vi "Teleop.vi"(10 "Match Info":T1={"Autonomous Elapsed Seconds"=0.0, "TeleOp Elapsed Seconds"=0.0, "Disabled Elapsed Seconds"=0.0, "Visited Autonomous"=FALSE, "Visited TeleOp"=FALSE, "Visited Disabled"=FALSE, "Autonomous Settings"={"Autonomous Style"=enum."Independent", "VI Refnum"=refnum}}, 11 "Call Context":T2) -> ()   [LabVIEW 2015]
doc: "This VI is called for each TeleOp packet received from the DS where the robot is not disabled. It is often used to read from the joysticks and update I/O or to update setpoints for timed control loops. It should complete and return within 20 milliseconds or it may miss DS packets."
uses:
  <vilib>/Rock Robotics/WPI/DriverStation/WPI_DriverStationDerivedRobotMode.ctl
  <vilib>/Rock Robotics/WPI/DriverStation/WPI_DriverStationMatch Info.ctl
  <vilib>/Rock Robotics/WPI/Utilities/WPI_GetSetVariantRefNum.vi
  <vilib>/Rock Robotics/Network Tables/NT Write Numeric Array.vi
  <vilib>/Rock Robotics/Network Tables/NT Read Boolean.vi
  <vilib>/Rock Robotics/Network Tables/NT Write Boolean.vi
  <vilib>/Rock Robotics/Network Tables/NT Write Number.vi
  <vilib>/Rock Robotics/Network Tables/NT Read Number.vi
  <vilib>/Rock Robotics/Network Tables/NT Write Boolean Array.vi
panel:
  out "Low Switch":bool
  out "High Switch":bool
  out "POT Sensor Meter":dbl(knob) scale=78.0..98.0
  out "POT Sensor Value":dbl
  out "Sample Slider 0":dbl(slide) scale=0.0..5.0
  out "Sample Boolean 1":bool
  out "Sample Boolean 0":bool
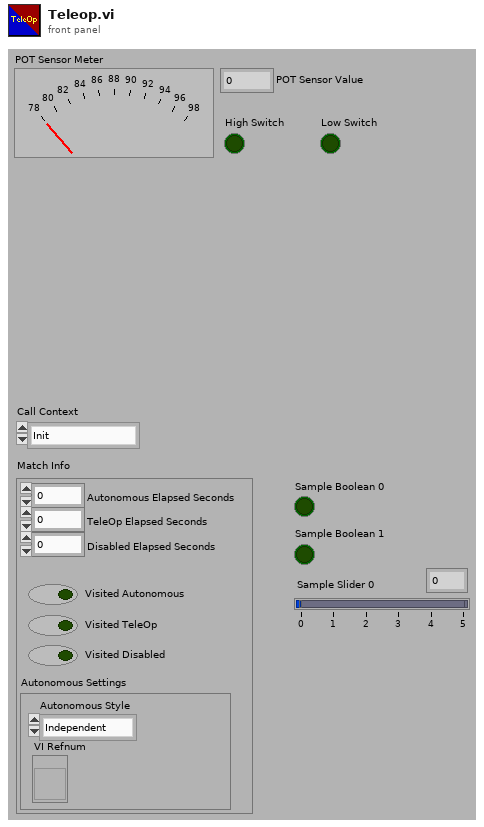
[diagram p1: front panel]
types:
  T1 = typedef "WPI_DriverStationMatch Info.ctl" = cluster{"Autonomous Elapsed Seconds":dbl, "TeleOp Elapsed Seconds":dbl, "Disabled Elapsed Seconds":dbl, "Visited Autonomous":bool, "Visited TeleOp":bool, "Visited Disabled":bool, "Autonomous Settings":cluster{"Autonomous Style":enum16{"Iterative", "Independent"}, "VI Refnum":refnum<vi>}}
  T2 = typedef "WPI_DriverStationDerivedRobotMode.ctl" = enum16{"Init", "Execute", "Stop"}
  T3 = typedef "WPI_JoystickDevRef.ctl" = cluster{"Device":T4}
  T4 = typedef "WPI_JoystickDeviceEnum.ctl" = enum16{"USB 0", "USB 1", "USB 2", "USB 3", "USB 4", "USB 5"}
  T5 = typedef "WPI_SwitchDevRef.ctl" = cluster{"DevStatus":errorcluster, "DIO Channel":T6, "CntIndex":T7, "Normally Closed":bool}
  T6 = typedef "FPGA_DIOChannel.ctl" = enum8{"DIO 0", "DIO 1", "DIO 2", "DIO 3", "DIO 4", "DIO 5", "DIO 6", "DIO 7", "DIO 8", "DIO 9", "DIO MXP 0", "DIO MXP 1", "DIO MXP 2", "DIO MXP 3", "DIO MXP 4", "DIO MXP 5", "DIO MXP 6", "DIO MXP 7", "DIO MXP 8", "DIO MXP 9", "DIO MXP 10", "DIO MXP 11", "DIO MXP 12", "DIO MXP 13", "DIO MXP 14", "DIO MXP 15", "Invalid"}
  T7 = typedef "FPGA_CounterCtrSystemIndex.ctl" = enum8{"Ctr 0", "Ctr 1", "Ctr 2", "Ctr 3", "Ctr 4", "Ctr 5", "Ctr 6", "Ctr 7", "Invalid"}
  T8 = typedef "WPI_PotentiometerDevRef.ctl" = cluster{"DevStatus":errorcluster, "Analog Channel":T9, "Invert Output":bool}
  T9 = typedef "FPGA_AIChannel.ctl" = enum8{"AI 0", "AI 1", "AI 2", "AI 3", "AI MXP 0", "AI MXP 1", "AI MXP 2", "AI MXP 3", "Invalid"}
  T10 = cluster{"Axes[0]":dbl, "Axes[1]":dbl, "Axes[2]":dbl, "Axes[3]":dbl, "Axes[4]":dbl, "Axes[5]":dbl, "Axes[6]":dbl, "Axes[7]":dbl, "Axes[8]":dbl}
  T11 = typedef "WPI_RobotDriveDevRef.ctl" = cluster{"DevStatus":errorcluster, "Motors[]":T12[], "Square Inputs":bool, "Max Output":dbl}
  T12 = typedef "WPI_MotorControlDeviceRef.ctl" = cluster{"DeviceStatus":errorcluster, "Type":T13, "PWM":cluster{"PWM Channel":T14, "DeadBand":T15}, "CAN":cluster{"Device Number":u8, "Control Mode":T16, "Semaphore":T17, "Max Vout":dbl, "TalonSRX Control Mode":T18}, "Invert":bool}
  T13 = typedef "WPI_MotorControlType.ctl" = enum16{"PWM", "CAN", "CANTalonSRX"}
  T14 = typedef "FPGA_DIOPWMChannel.ctl" = enum8{"PWM 0", "PWM 1", "PWM 2", "PWM 3", "PWM 4", "PWM 5", "PWM 6", "PWM 7", "PWM 8", "PWM 9", "PWM MXP 0", "PWM MXP 1", "PWM MXP 2", "PWM MXP 3", "PWM MXP 4", "PWM MXP 5", "PWM MXP 6", "PWM MXP 7", "PWM MXP 8", "PWM MXP 9", "Invalid"}
  T15 = typedef "WPI_PWMDeadband.ctl" = cluster{"Name":string, "maxPositivePwm":i32, "minPositivePwm":i32, "centerPwm":i32, "maxNegativePwm":i32, "minNegativePwm":i32, "angularRange":u16}
  T16 = typedef "WPI_CANJaguar_ControlMode.ctl" = enum8{"Percent VBus", "Current", "Speed", "Position", "Voltage"}
  T17 = typedef "Semaphore RefNum" = refnum<k1>
  T18 = typedef "WPI_CANTalonSRX_APIControlMode.ctl" = enum8{"Percent VBus", "Speed", "Position", "Slave", "Unchanged / Invalid", "Voltage Compensation", "Current", "Motion Profile"}
  T19 = cluster{"Buttons[0]":bool, "Buttons[1]":bool, "Buttons[2]":bool, "Buttons[3]":bool, "Buttons[4]":bool, "Buttons[5]":bool, "Buttons[6]":bool, "Buttons[7]":bool, "Buttons[8]":bool}
  T20 = typedef "WPI_ServoDeviceRef.ctl" = cluster{"DeviceStatus":errorcluster, "PWM Channel":T14, "DeadBand":T15}
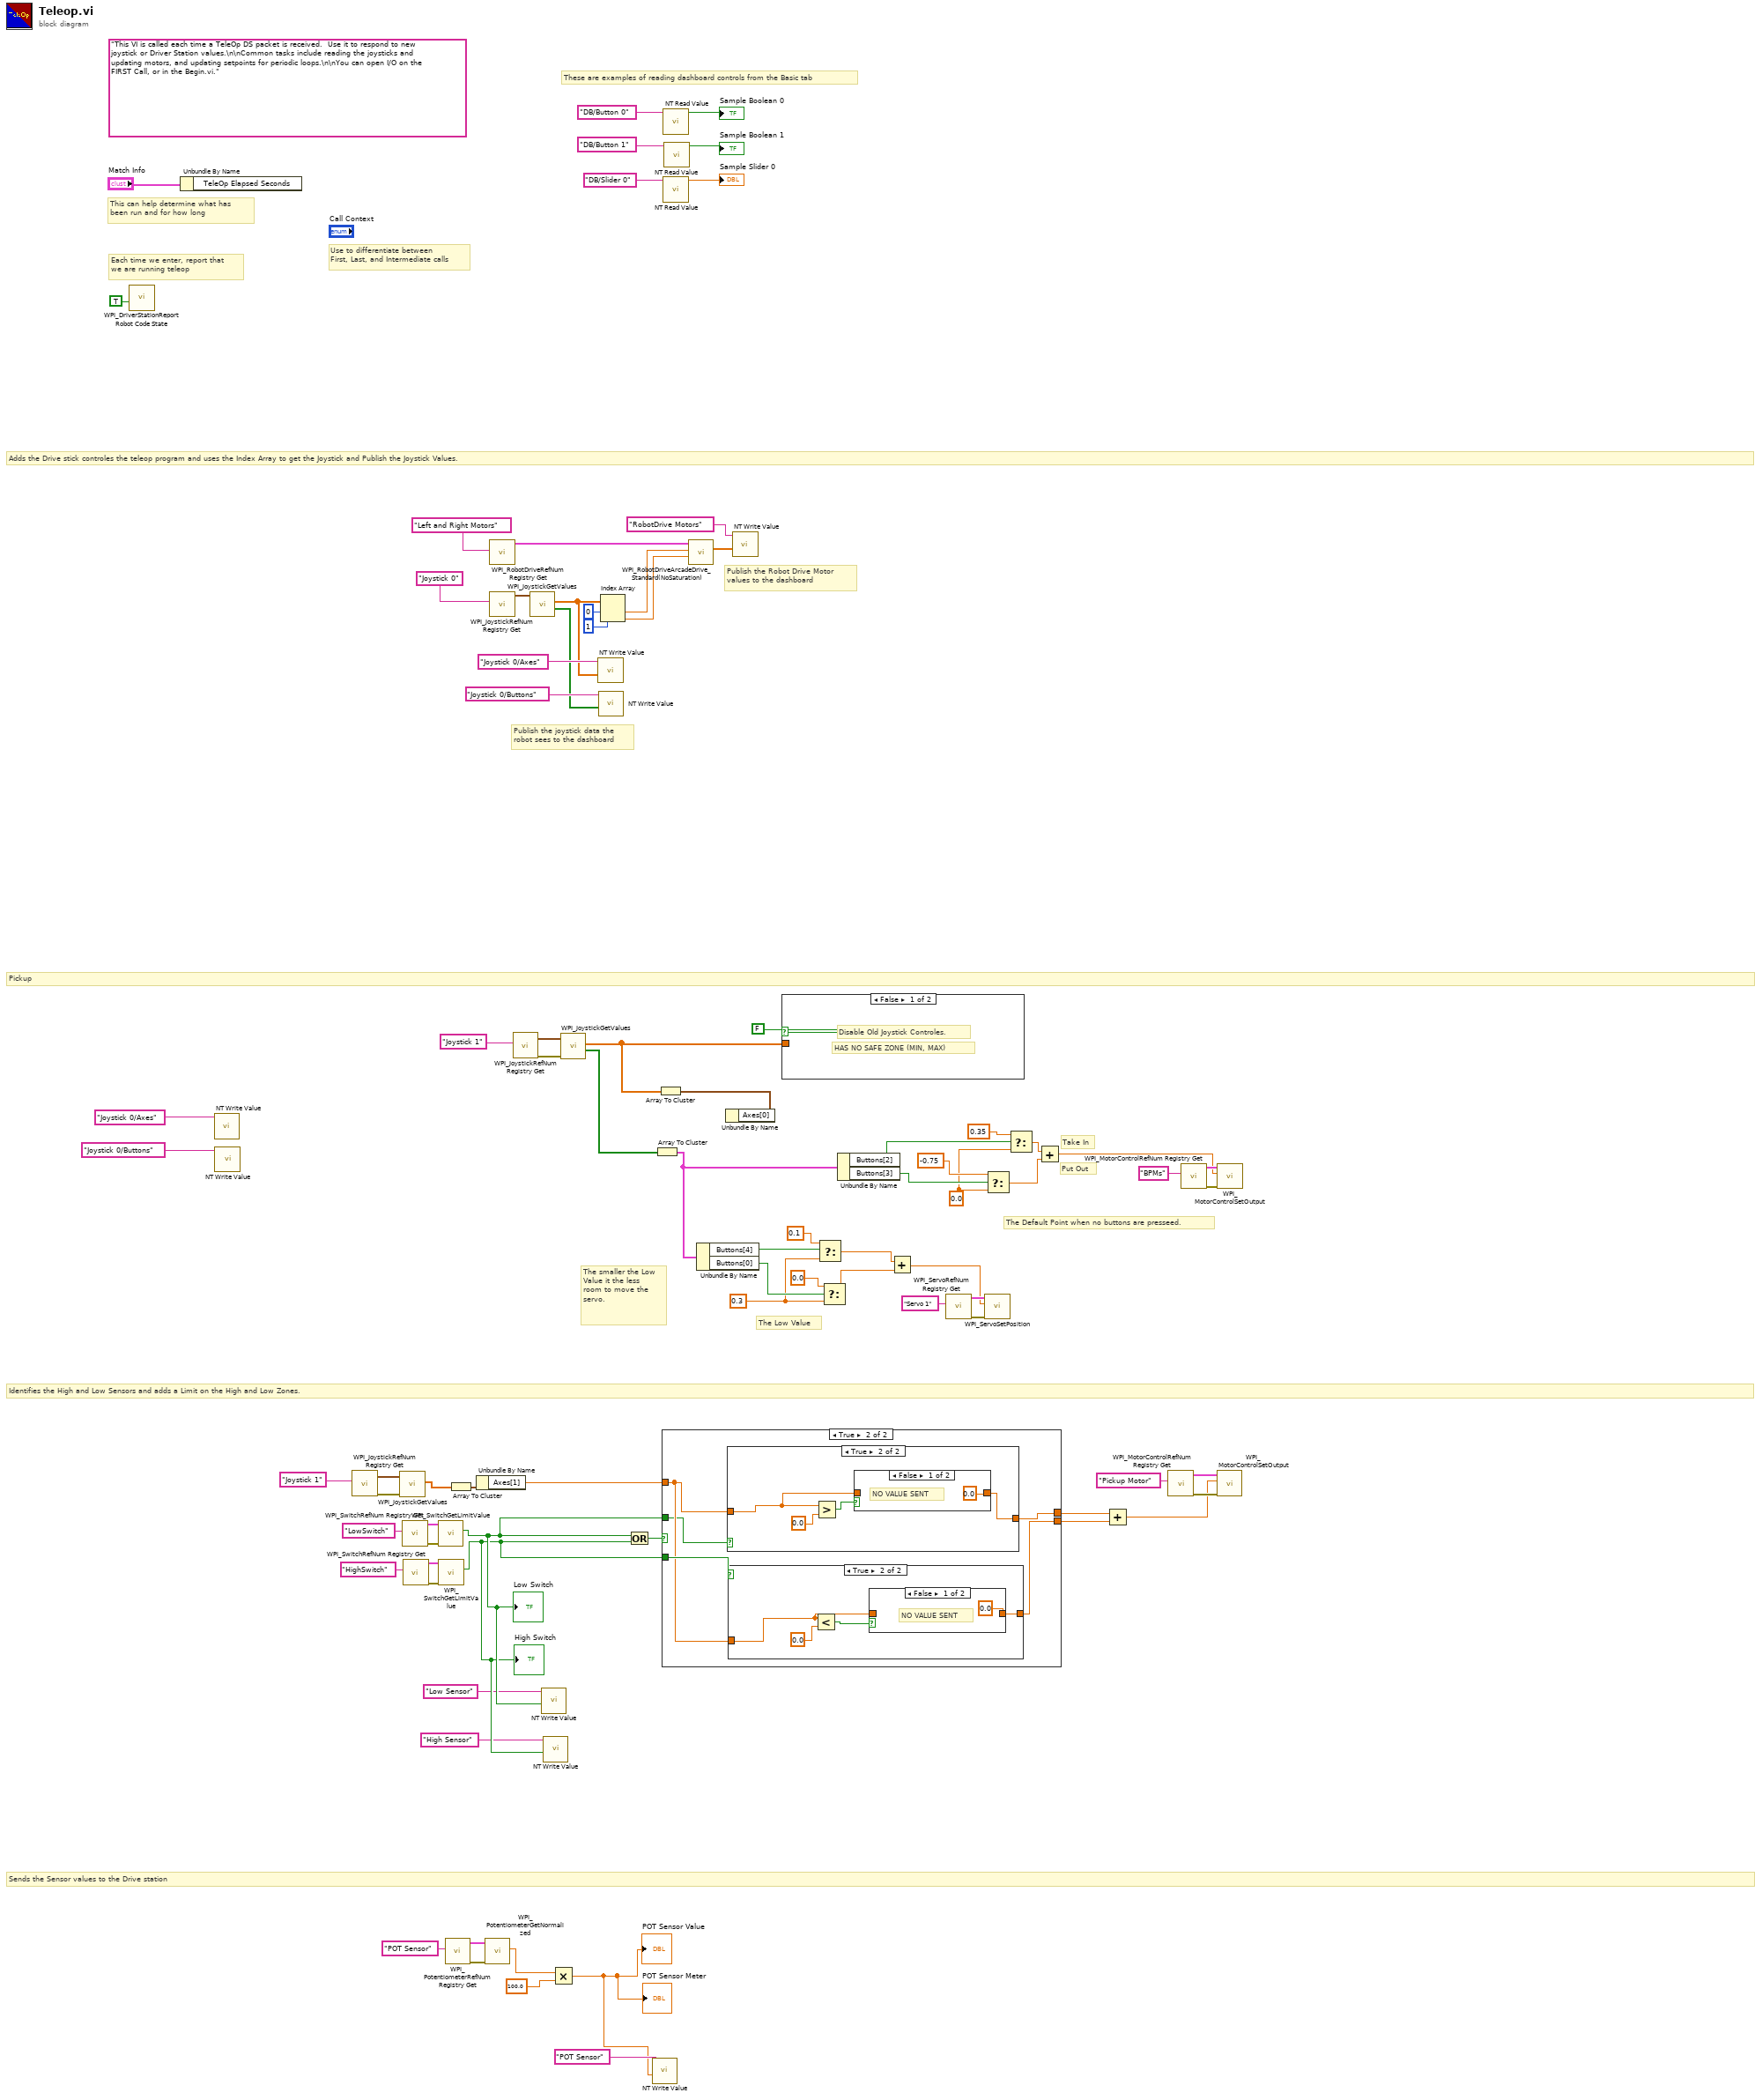
[diagram p0: block diagram]
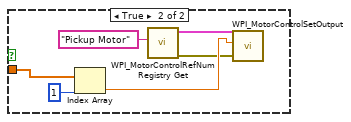
[diagram p2: hidden frame]
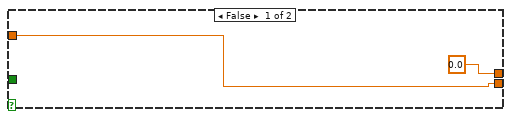
[diagram p3: hidden frame]
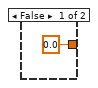
[diagram p4: hidden frame]
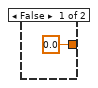
[diagram p6: hidden frame]
diagram:
  w3 = 0.3 ("f")
  w1 = 0.0 ("f")
  (unwired) "This VI is called each time a TeleOp DS packet is received.  Use it to respond to new joystick or Driver Station values.\n\nCommon tasks include reading the joysticks and updating motors, and updating setpoints for periodic loops.\n\nYou can open I/O on the FIRST Call, or in the Begin.vi."
  # "Adds the Drive stick controles the teleop program and uses the Index Array to get the Joystick and Publish the Joystick Values."
  # "Sends the Sensor values to the Drive station"
  # "Identifies the High and Low Sensors and adds a Limit on the High and Low Zones."
  # "The Default Point when no buttons are presseed."
  # "The smaller the Low Value it the less room to move the servo."
  # "The Low Value"
  # "Put Out"
  # "Take In"
  # "Pickup"
  # "These are examples of reading dashboard controls from the Basic tab"
  # "Publish the Robot Drive Motor\nvalues to the dashboard"
  # "Publish the joystick data the\nrobot sees to the dashboard"
  # "Each time we enter, report that\nwe are running teleop"
  # "Use to differentiate between\nFirst, Last, and Intermediate calls"
  # "This can help determine what has\nbeen run and for how long"
  n1 = call <vilib>:"WPI_DriverStationReport Robot Code State.vi"("TeleOp"=TRUE ("Autonomous")) -> ()  [unwired: 10 in, 1 out]
  n2 = Unbundle By Name("Match Info") -> ()  [unwired: 1 out]
  n3 = call-poly <vilib>:"NT Write Value.vi"("Name"="Joystick 0/Axes") -> ()  [unwired: 10 in, 1 out]
  n4 = call-poly <vilib>:"NT Write Value.vi"("Name"="Joystick 0/Buttons") -> ()  [unwired: 10 in, 1 out]
  n5 = call <vilib>:"WPI_JoystickRefNum Registry Get.vi"("refnum name"="Joystick 1") -> ("error out"=w37:errorcluster, "JoystickDevRef"=w38:T3)  [unwired: 9 in]
  n6 = call <vilib>:"WPI_JoystickGetValues.vi"("error in (no error)"=w37, "JoystickDevRef"=w38) -> ("Axes"=w36:dbl[])  [unwired: 5 in, 4 out]
  n7 = call <vilib>:"WPI_SwitchRefNum Registry Get.vi"("refnum name"="LowSwitch") -> ("error out"=w44:errorcluster, "SwitchDevRef"=w45:T5)  [unwired: 9 in]
  n8 = call <vilib>:"WPI_SwitchRefNum Registry Get.vi"("refnum name"="HighSwitch") -> ("error out"=w41:errorcluster, "SwitchDevRef"=w42:T5)  [unwired: 9 in]
  n9 = call <vilib>:"WPI_SwitchGetLimitValue.vi"("error in (no error)"=w44, "SwitchDevRef"=w45) -> ("Switch Pressed"=w21:bool)  [unwired: 7 in, 2 out]
  "Low Switch" <- w21
  n10 = call <vilib>:"WPI_SwitchGetLimitValue.vi"("error in (no error)"=w41, "SwitchDevRef"=w42) -> ("Switch Pressed"=w20:bool)  [unwired: 7 in, 2 out]
  "High Switch" <- w20
  n11 = call <vilib>:"WPI_PotentiometerRefNum Registry Get.vi"("refnum name"="POT Sensor") -> ("error out"=w25:errorcluster, "PotDevRef"=w24:T8)  [unwired: 9 in]
  n12 = Array To Cluster(array=w36) -> (cluster=w35:T10)
  n13 = Unbundle By Name(w35) -> ("Axes[1]"=w34:dbl)
  n14 = call <vilib>:"WPI_PotentiometerGetNormalized.vi"("error in"=w25, "PotDevRef"=w24) -> ("Normalized Value"=w17:dbl)  [unwired: 7 in, 2 out]
  n15 = call <vilib>:"WPI_RobotDriveRefNum Registry Get.vi"("refnum name"="Left and Right Motors") -> ("RobotDriveDevRef"=w82:T11)  [unwired: 1 in, 9 out]
  n16 = call <vilib>:"WPI_JoystickRefNum Registry Get.vi"("refnum name"="Joystick 0") -> ("JoystickDevRef"=w79:T3)  [unwired: 1 in, 9 out]
  n17 = call <vilib>:"WPI_JoystickRefNum Registry Get.vi"("refnum name"="Joystick 1") -> ("error out"=w61:errorcluster, "JoystickDevRef"=w62:T3)  [unwired: 9 in]
  n18 = call <vilib>:"WPI_JoystickGetValues.vi"("JoystickDevRef"=w79) -> ("Buttons"=w47:bool[], "Axes"=w74:dbl[])  [unwired: 6 in, 3 out]
  n19 = call-poly <vilib>:"NT Write Value.vi"("Boolean"=w21, "Name"="Low Sensor") -> ()  [unwired: 9 in, 1 out]
  n20 = call-poly <vilib>:"NT Write Value.vi"("Boolean"=w20, "Name"="High Sensor") -> ()  [unwired: 9 in, 1 out]
  n21 = Multiply(x=w17, y=100.0) -> (x*y=w15:dbl)
  "POT Sensor Value" <- w15
  "POT Sensor Meter" <- w15
  n22 = call <vilib>:"WPI_JoystickGetValues.vi"("error in (no error)"=w61, "JoystickDevRef"=w62) -> ("Buttons"=w50:bool[], "Axes"=w26:dbl[])  [unwired: 5 in, 3 out]
  n23 = call-poly <vilib>:"NT Write Value.vi"("Numeric Array"=w74, "Name"="Joystick 0/Axes") -> ()  [unwired: 9 in, 1 out]
  n24 = call-poly <vilib>:"NT Write Value.vi"("Boolean Array"=w47, "Name"="Joystick 0/Buttons") -> ()  [unwired: 9 in, 1 out]
  n25 = Index Array(array=w74, index #1=0 ("index"), index #2=1 ("index")) -> (element #1=w81:dbl, element #2=w77:dbl)
  n26 = Or(x=w21, y=w20) -> (x .or. y?=w46:bool)
  n27 = call-poly <vilib>:"NT Write Value.vi"("Numeric"=w15, "Name"="POT Sensor") -> ()  [unwired: 9 in, 1 out]
  n28 = Array To Cluster(array=w50) -> (cluster=w5:T19)
  n29 = Array To Cluster(array=w26) -> (cluster=w49:T10)
  n30 = case shown="True" w46 {
    tunnel: w21 -> [_ w89]
    tunnel: w20 -> [_ w91]
    tunnel: w34 -> [w85 w90]
    tunnel: [0.0 ("Axes[1]") w88] -> w29
    tunnel: [w85 w87] -> w28
    frame False {
    }
    frame True {
      n31 = case shown="True" w89 {
        tunnel: w90 -> [_ w101]
        tunnel: [0.0 ("Axes[1]") w100] -> w88
        frame False {
        }
        frame True {
          n32 = Greater?(x=w101, y=0.0) -> (0:w102:bool)
          n33 = case shown="False" w102 {
            tunnel: [0.0 ("Axes[1]") w105] -> w100
            tunnel: w101 -> [_ w105]
            frame False {
              # "NO VALUE SENT"
            }
            frame True {
            }
          }
        }
      }
      n34 = case shown="True" w91 {
        tunnel: w90 -> [_ w93]
        tunnel: [0.0 ("Axes[1]") w94] -> w87
        frame False {
        }
        frame True {
          n35 = Less?(x=w93, y=0.0) -> (x < y?=w95:bool)
          n36 = case shown="False" w95 {
            tunnel: [0.0 ("Axes[1]") w98] -> w94
            tunnel: w93 -> [_ w98]
            frame False {
              # "NO VALUE SENT"
            }
            frame True {
            }
          }
        }
      }
    }
  }
  n37 = call-poly <vilib>:"NT Read Value.vi"("Name"="DB/Button 0" ("refnum name")) -> ("Boolean"=→"Sample Boolean 0":bool)  [unwired: 9 in, 1 out]
  n38 = call-poly <vilib>:"NT Read Value.vi"("Name"="DB/Slider 0" ("refnum name")) -> ("Numeric"=→"Sample Slider 0":dbl)  [unwired: 9 in, 1 out]
  n39 = call-poly <vilib>:"NT Read Value.vi"("Name"="DB/Button 1" ("refnum name")) -> ("Boolean"=→"Sample Boolean 1":bool)  [unwired: 9 in, 1 out]
  n40 = call <vilib>:"WPI_RobotDriveArcadeDrive_Standard(NoSaturation).vi"("Y axis value"=w77, "X axis value"=w81, "RobotDriveDevRef"=w82) -> ("Motor Values"=w67:dbl[])  [unwired: 1 in, 7 out]
  n41 = Unbundle By Name(w5) -> ("Buttons[4]"=w4:bool, "Buttons[0]"=w9:bool)
  n42 = Unbundle By Name(w49) -> ()  [unwired: 1 out]
  n43 = call-poly <vilib>:"NT Write Value.vi"("Numeric Array"=w67, "Name"="RobotDrive Motors") -> ()  [unwired: 9 in, 1 out]
  n44 = case shown="False" FALSE {
    tunnel: w26 -> [_ w106]
    frame False {
      # "HAS NO SAFE ZONE (MIN, MAX)"
      # "Disable Old Joystick Controles."
    }
    frame True {
      n45 = Index Array(array=w106, index=1) -> (element=w110:dbl)
      n46 = call <vilib>:"WPI_MotorControlRefNum Registry Get.vi"("refnum name"="Pickup Motor") -> ("error out"=w107:errorcluster, "MotorControlDevRef"=w108:T12)  [unwired: 9 in]
      n47 = call <vilib>:"WPI_MotorControlSetOutput.vi"("error in (no error)"=w107, "Output"=w110, "MotorControlDevRef"=w108) -> ()  [unwired: 6 in, 3 out]
    }
  }
  n48 = Select(t=0.1, s=w4, f=w3) -> (s? t:f=w6:dbl)
  n49 = Select(t=0.0, s=w9, f=w3) -> (s? t:f=w8:dbl)
  n50 = Unbundle By Name(w5) -> ("Buttons[2]"=w48:bool, "Buttons[3]"=w2:bool)
  n51 = Add(x=w6, y=w8) -> (x+y=w7:dbl)
  n52 = call <vilib>:"WPI_ServoRefNum Registry Get.vi"("refnum name"="Servo 1") -> ("error out"=w13:errorcluster, "ServoDeviceRef"=w12:T20)  [unwired: 9 in]
  n53 = call <vilib>:"WPI_ServoSetPosition.vi"("error in (no error)"=w13, "Position"=w7, "ServoDeviceRef"=w12) -> ()  [unwired: 7 in, 2 out]
  n54 = Select(t=-0.75, s=w2, f=w1) -> (s? t:f=w54:dbl)
  n55 = Select(t=0.35, s=w48, f=w1) -> (s? t:f=w55:dbl)
  n56 = Add(x=w55, y=w54) -> (x+y=w53:dbl)
  n57 = Add(x=w29, y=w28) -> (x+y=w30:dbl)
  n58 = call <vilib>:"WPI_MotorControlRefNum Registry Get.vi"("refnum name"="Pickup Motor") -> ("error out"=w33:errorcluster, "MotorControlDevRef"=w32:T12)  [unwired: 9 in]
  n59 = call <vilib>:"WPI_MotorControlRefNum Registry Get.vi"("refnum name"="BPMs") -> ("error out"=w59:errorcluster, "MotorControlDevRef"=w60:T12)  [unwired: 9 in]
  n60 = call <vilib>:"WPI_MotorControlSetOutput.vi"("error in (no error)"=w33, "Output"=w30, "MotorControlDevRef"=w32) -> ()  [unwired: 6 in, 3 out]
  n61 = call <vilib>:"WPI_MotorControlSetOutput.vi"("error in (no error)"=w59, "Output"=w53, "MotorControlDevRef"=w60) -> ()  [unwired: 6 in, 3 out]
